vi "timestamp.vi"() -> ()   [LabVIEW 2017]
panel:
  in  "stop 2":bool
  out "Shift":string
  out "time string":string
  in  "stop":bool
  out "Waveform Chart":dbl(graph)
  in  "error in (no error)":errorcluster
  out "error out":errorcluster
  out "Boolean 2":bool
  out "Boolean":bool
  out "number (0 to 1)":dbl
  out "Present (s)":dbl
  out "Elapsed Time (s)":dbl
  out "Elapsed Time Text":string
  out "error out 2":errorcluster
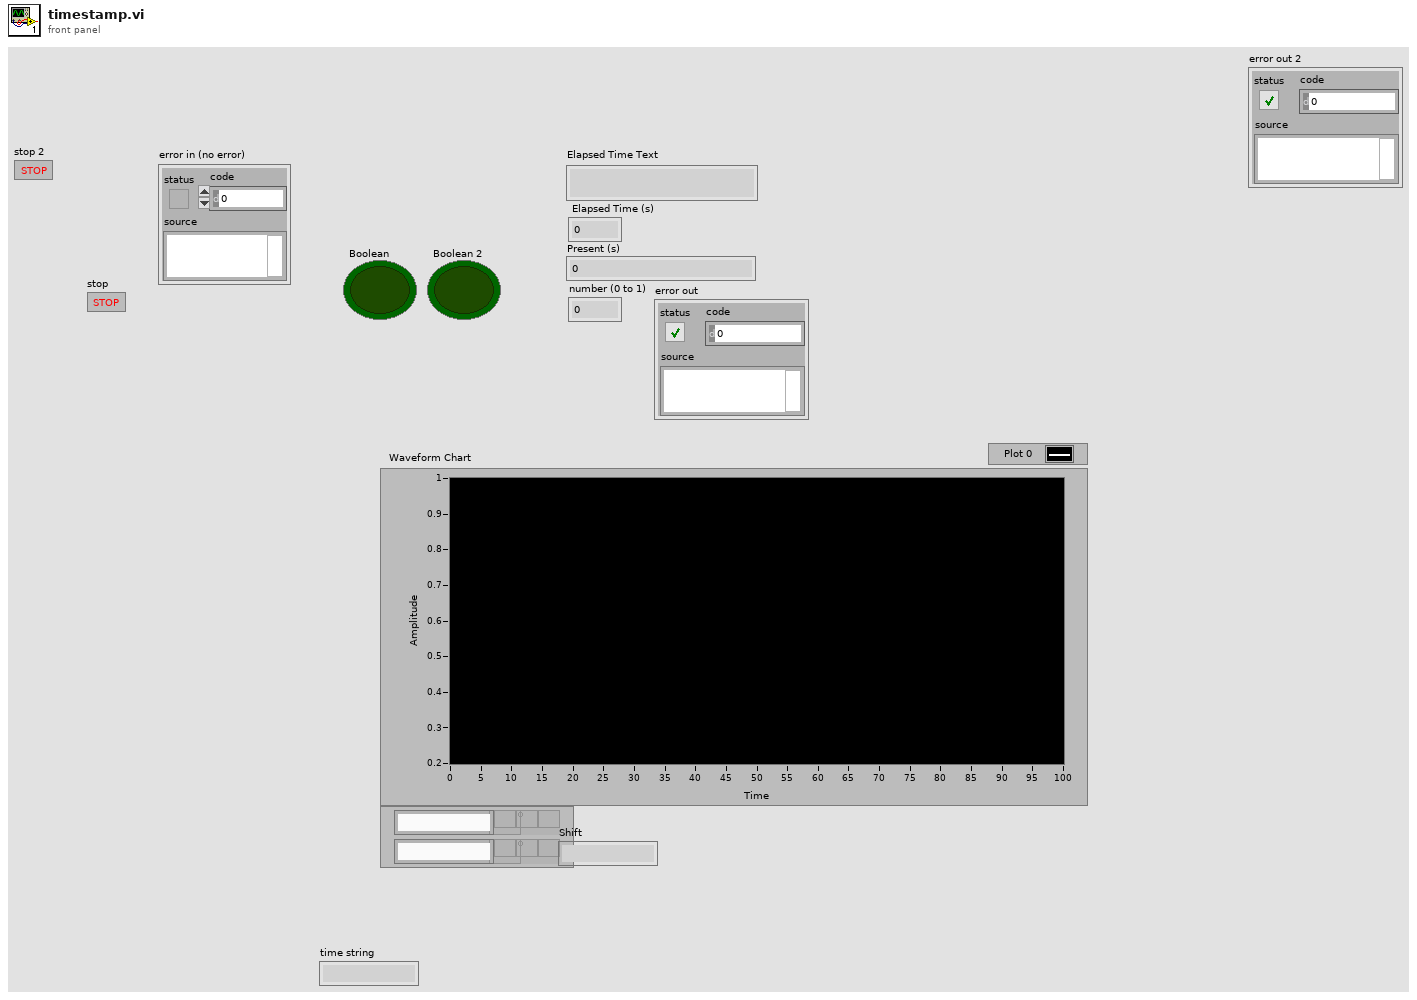
[diagram p1: front panel]
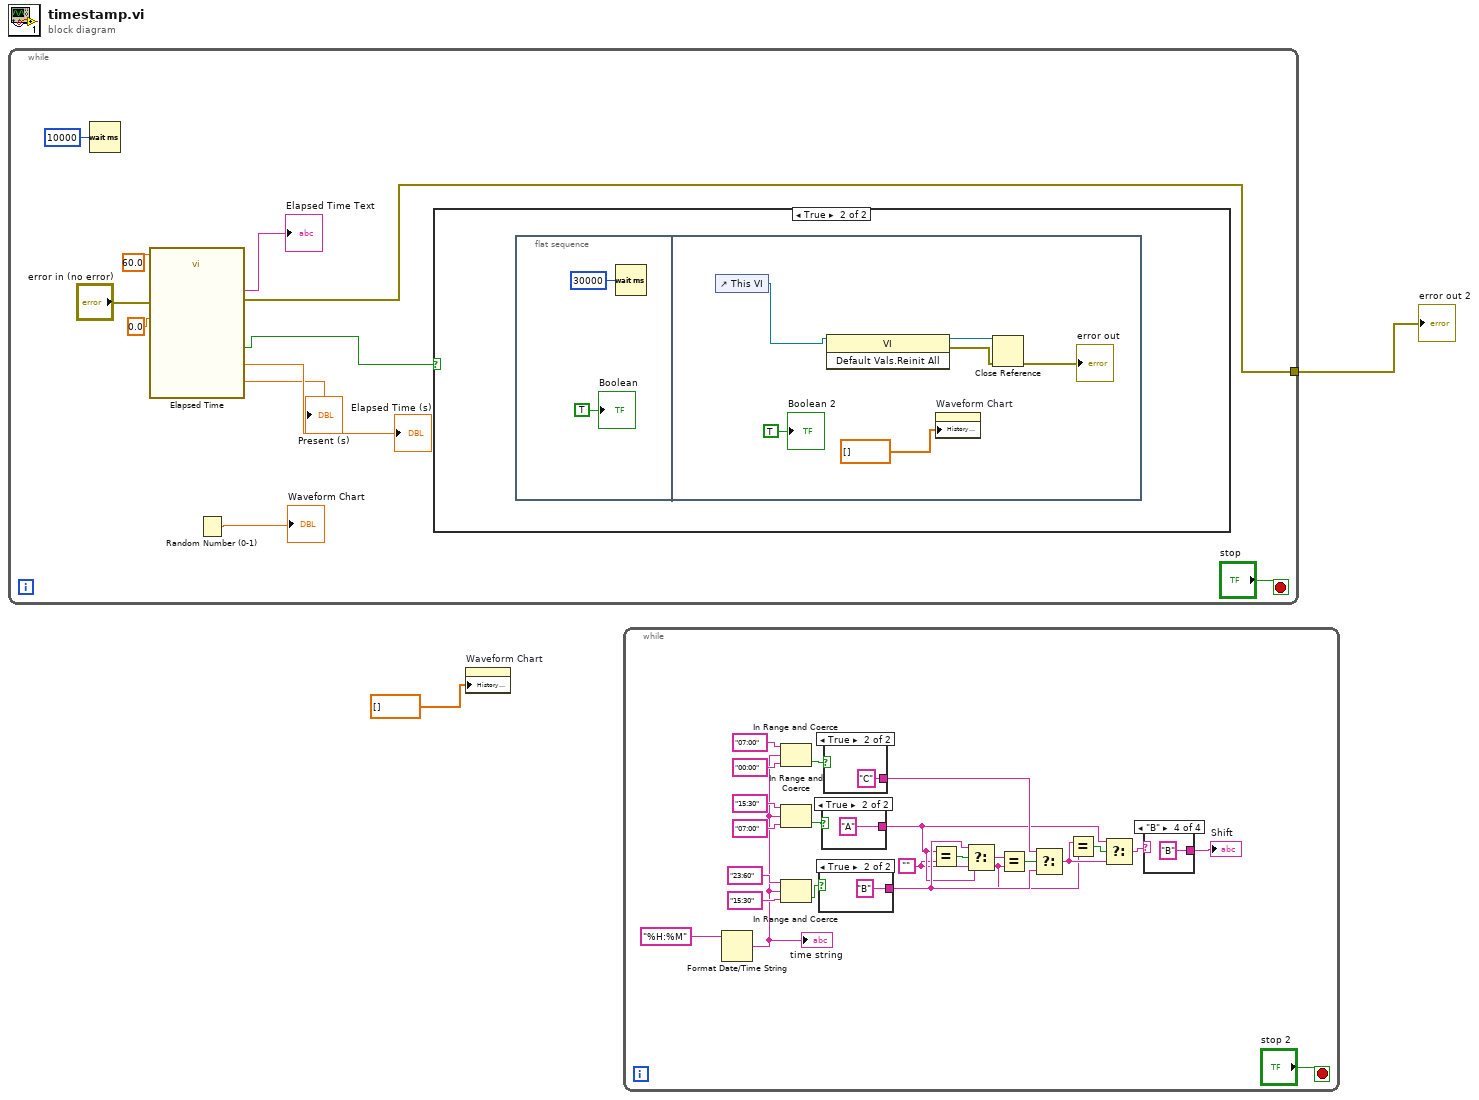
[diagram p0: block diagram]
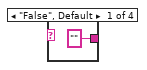
[diagram p2: hidden frame]
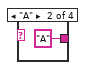
[diagram p3: hidden frame]
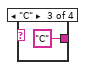
[diagram p4: hidden frame]
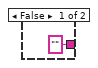
[diagram p5: hidden frame]
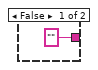
[diagram p6: hidden frame]
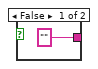
[diagram p7: hidden frame]
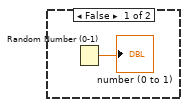
[diagram p8: hidden frame]
diagram:
  n1 = while {
    tunnel: [w6] -> w2
    stop <- "stop" stop-if-true
    n2 = Wait (ms)(milliseconds to wait=u32 10000) -> ()  [unwired: 1 out]
    n3 = call "Elapsed Time"("Time Target (s)"=60.0, "error in (no error)"="error in (no error)", "Set Start Time (s)"=0.0) -> ("Present (s)"=→"Present (s)":dbl, "Elapsed Time (s)"=→"Elapsed Time (s)":dbl, "Time has Elapsed"=w8:bool, "Elapsed Time Text"=→"Elapsed Time Text":string, "error out"=w6:errorcluster)  [unwired: 9 in, 3 out]
    n4 = Random Number (0-1)() -> (number: 0 to 1=→"Waveform Chart":dbl)
    n5 = case shown="True" w8 {
      frame False {
        n6 = Random Number (0-1)() -> (number: 0 to 1=→"number (0 to 1)":dbl)
      }
      frame True {
        n7 = flat-sequence {
          frame #0 {
            n8 = Wait (ms)(milliseconds to wait=u32 30000) -> ()  [unwired: 1 out]
            "Boolean" <- TRUE ("Boolean")
          }
          frame #1 {
            n9 = control-ref of="This VI"() -> (w18:refnum<vi>)
            n10 = invoke class="VI" method="Default Vals.Reinit All"(reference=w18) -> (reference out=w21:refnum<vi>, error out=w22:errorcluster)  [unwired: 2 in, 1 out]
            n11 = property on="Waveform Chart" class="WFChart (strict)"("History Data"=dbl[] []) -> ()  [unwired: 2 in, 2 out]
            n12 = Close Reference(reference=w21, error in (no error)=w22) -> (error out=→"error out":errorcluster)
            "Boolean 2" <- TRUE ("Boolean 2")
          }
        }
      }
    }
  }
  "error out 2" <- w2
  n13 = property on="Waveform Chart" class="WFChart (strict)"("History Data"=dbl[] []) -> ()  [unwired: 2 in, 2 out]
  n14 = while {
    stop <- "stop 2" stop-if-true
    w27 = ""
    n15 = Format Date/Time String(time format string (%c)="%H:%M") -> (date/time string=w24:string)  [unwired: 2 in]
    "time string" <- w24
    n16 = In Range and Coerce(upper limit="07:00" ("String"), x=w24, lower limit="00:00" ("String")) -> (In Range?=w37:bool)  [unwired: 1 out]
    n17 = In Range and Coerce(upper limit="15:30" ("String"), x=w24, lower limit="07:00" ("String")) -> (In Range?=w43:bool)  [unwired: 1 out]
    n18 = In Range and Coerce(upper limit="23:60" ("String"), x=w24, lower limit="15:30" ("String")) -> (In Range?=w40:bool)  [unwired: 1 out]
    n19 = case shown="True" w40 {
      tunnel: ["" ("String") "B" ("String")] -> w32
      frame False {
      }
      frame True {
      }
    }
    n20 = case shown="True" w43 {
      tunnel: ["" ("String") "A" ("String")] -> w30
      frame False {
      }
      frame True {
      }
    }
    n21 = case shown="True" w37 {
      tunnel: ["" ("String") "C" ("String")] -> w33
      frame False {
      }
      frame True {
      }
    }
    n22 = Equal?(x=w30, y=w27) -> (x = y?=w36:bool)
    n23 = Select(t=w32, s=w36, f=w30) -> (s? t:f=w35:string)
    n24 = Equal?(x=w35, y=w27) -> (x = y?=w34:bool)
    n25 = Select(t=w33, s=w34, f=w32) -> (s? t:f=w29:string)
    n26 = Equal?(x=w29, y=w27) -> (x = y?=w31:bool)
    n27 = Select(t=w30, s=w31, f=w29) -> (s? t:f=w28:string)
    n28 = case shown="\"B\"" w28 {
      tunnel: ["" ("String") "A" ("String") "C" ("String") "B" ("String")] -> w26
      frame "False", Default {
      }
      frame "A" {
      }
      frame "C" {
      }
      frame "B" {
      }
    }
    "Shift" <- w26
  }
